vi "VisionDashRead_FrontLeft.vi"() -> (0 "FL Ang Deg":dbl, 1 "FL Y Ft":dbl, 2 "FL X Ft":dbl, 3 "FL Error":bool, 4 "FL Time Sec":dbl, 5 "FL Conn":bool, 6 "FL Last Sec Cnt":i64, 7 "FL HasTarg":bool, 8 "FL Count":i64, 11 "FL NewData":bool)   [LabVIEW 2023]
doc: "Vision Network\n\nInput\n --Error in \n\nOutput\n --Error out"
uses:
  <vilib>/Rock Robotics/Network Tables/NT Read Integer.vi
  <vilib>/Rock Robotics/Network Tables/NT Read Boolean.vi
  <vilib>/Rock Robotics/Network Tables/NT Read Number.vi
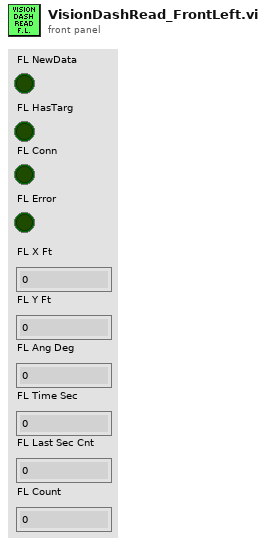
[diagram p1: front panel]
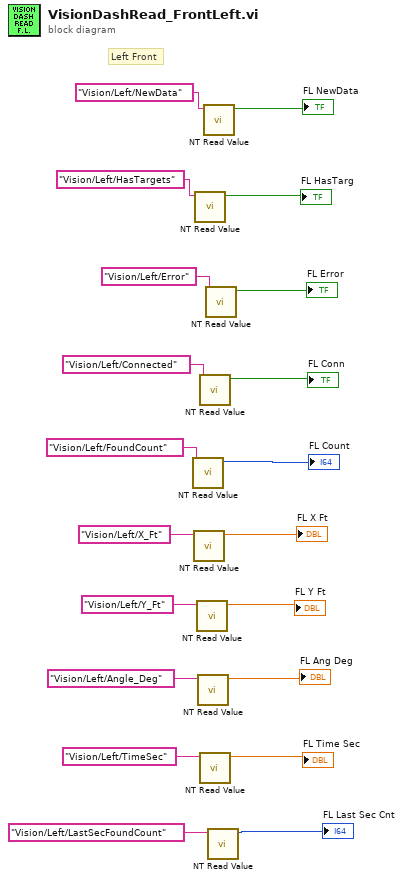
[diagram p0: block diagram]
diagram:
  # "Left Front"
  n1 = call-poly <vilib>:"NT Read Value.vi"("name"="Vision/Left/FoundCount") -> ("value"=→"FL Count":i64)  [unwired: 8 in, 2 out]
  n2 = call-poly <vilib>:"NT Read Value.vi"("name"="Vision/Left/X_Ft") -> ("value"=→"FL X Ft":dbl)  [unwired: 8 in, 2 out]
  n3 = call-poly <vilib>:"NT Read Value.vi"("name"="Vision/Left/HasTargets") -> ("value"=→"FL HasTarg":bool)  [unwired: 8 in, 2 out]
  n4 = call-poly <vilib>:"NT Read Value.vi"("name"="Vision/Left/Y_Ft") -> ("value"=→"FL Y Ft":dbl)  [unwired: 8 in, 2 out]
  n5 = call-poly <vilib>:"NT Read Value.vi"("name"="Vision/Left/Angle_Deg") -> ("value"=→"FL Ang Deg":dbl)  [unwired: 8 in, 2 out]
  n6 = call-poly <vilib>:"NT Read Value.vi"("name"="Vision/Left/Connected") -> ("value"=→"FL Conn":bool)  [unwired: 8 in, 2 out]
  n7 = call-poly <vilib>:"NT Read Value.vi"("name"="Vision/Left/TimeSec") -> ("value"=→"FL Time Sec":dbl)  [unwired: 8 in, 2 out]
  n8 = call-poly <vilib>:"NT Read Value.vi"("name"="Vision/Left/NewData") -> ("value"=→"FL NewData":bool)  [unwired: 8 in, 2 out]
  n9 = call-poly <vilib>:"NT Read Value.vi"("name"="Vision/Left/Error") -> ("value"=→"FL Error":bool)  [unwired: 8 in, 2 out]
  n10 = call-poly <vilib>:"NT Read Value.vi"("name"="Vision/Left/LastSecFoundCount") -> ("value"=→"FL Last Sec Cnt":i64)  [unwired: 8 in, 2 out]
